vi "Experiment log.vi"(8 "error in":errorcluster, 9 "file path (use dialog)":path, 10 "New experiment info (from Matlab)":string) -> (0 "error out":errorcluster, 3 "Experiment log out":string)   [LabVIEW 2017]
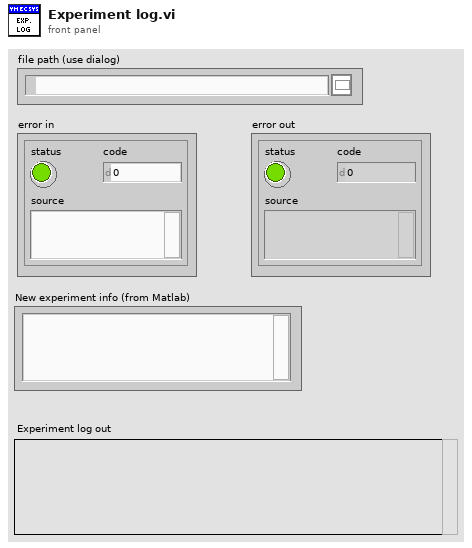
[diagram p1: front panel]
types:
  T1 = enum16{"open", "replace", "create", "open or create", "replace or create", "replace or create with confirmation"}
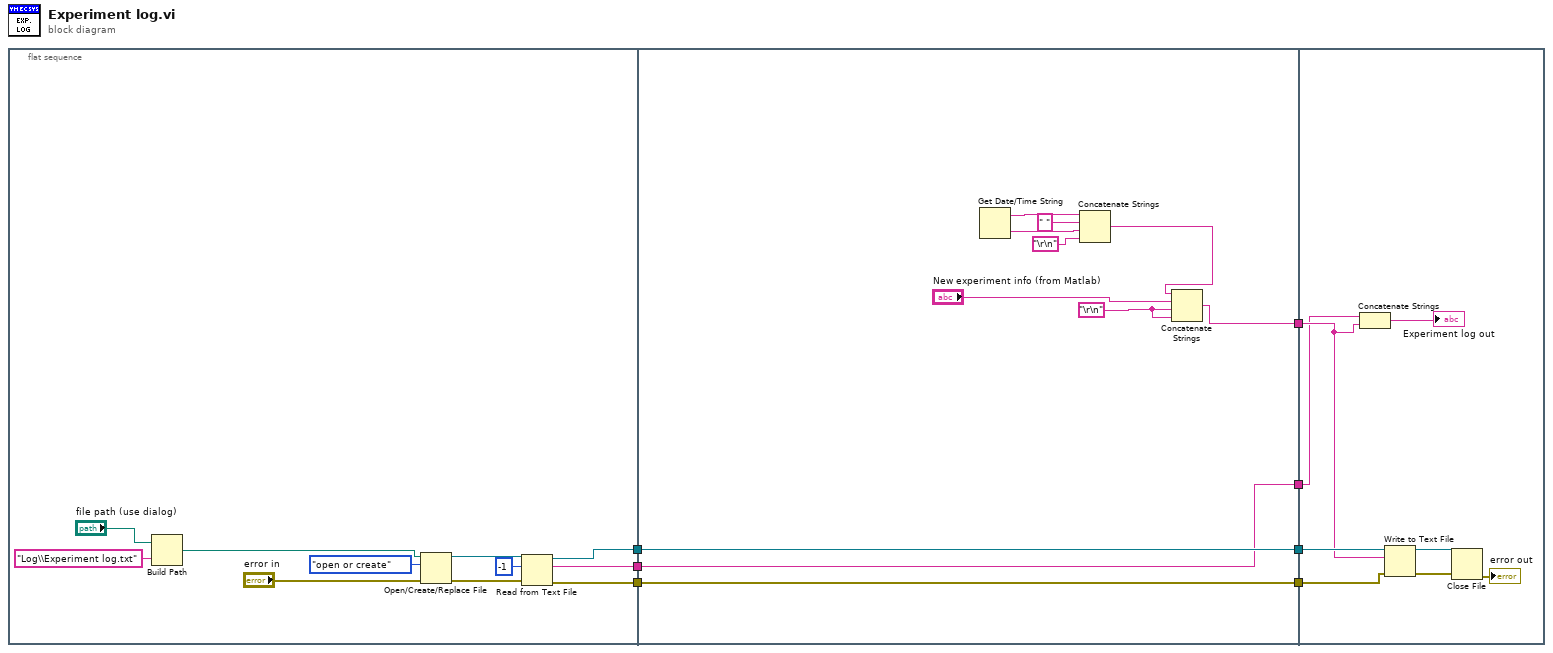
[diagram p0: block diagram]
diagram:
  n1 = flat-sequence {
    tunnel: [w12] -> w7
    tunnel: [w11] -> w6
    tunnel: [w10] -> w5
    tunnel: w7 -> [w21]
    tunnel: [w24] -> w4
    tunnel: w6 -> [w23]
    tunnel: [w23] -> w3
    tunnel: [w22] -> w2
    tunnel: w5 -> [w22]
    tunnel: [w21] -> w1
    tunnel: w4 -> [w31]
    tunnel: w3 -> [w37]
    tunnel: w2 -> [w36]
    tunnel: w1 -> [w30]
    frame #0 {
      n2 = Build Path(base path="file path (use dialog)", name or relative path="Log\\Experiment log.txt") -> (appended path=w8:path)
      n3 = Open/Create/Replace File(file path (use dialog)=w8, error in="error in", operation (0:open)=T1."open or create") -> (refnum out=w15:refnum<file>, error out=w14:errorcluster)  [unwired: 3 in, 1 out]
      n4 = Read from Text File(file (use dialog)=w15, count=-1, error in=w14) -> (refnum out=w11:refnum<file>, text=w12:string, error out=w10:errorcluster)  [unwired: 1 in, 1 out]
    }
    frame #1 {
      w19 = "\r\n"
      n5 = Get Date/Time String() -> (date string=w29:string, time string=w27:string)  [unwired: 3 in]
      n6 = Concatenate Strings(w29, " " ("string"), w27, "\r\n") -> (w25:string)
      n7 = Concatenate Strings(w25, "New experiment info (from Matlab)", w19, w19) -> (w24:string)
    }
    frame #2 {
      n8 = Concatenate Strings(w30, w31) -> (→"Experiment log out":string)
      n9 = Write to Text File(file (use dialog)=w37, text=w31, error in=w36) -> (refnum out=w35:refnum<file>, error out=w34:errorcluster)  [unwired: 1 in, 1 out]
      n10 = Close File(refnum=w35, error in=w34) -> (error out=→"error out":errorcluster)  [unwired: 1 out]
    }
  }
